vi "5. CSM Data Type.vi"() -> ()   [LabVIEW 2017]
doc: "### 5. CSM Data Type.vi\n\n#### Overview\n\nDemonstrates the data type descriptions recommended by CSM.\n\n#### Introduction\n\nIn the CSM framework, arguments can only be passed in the form of String types. To support various data types, data usually needs to go through a process of packing, transmission, and unpacking. For example, CSM internally provides support for the HEXSTR argument type, and users can also provide custom data type conversions via addons to suit their application scenarios.\n\nTo support different data types, you sometimes need to pass data type descriptions to handle logic branches for different data types at the decoding stage. This example demonstrates the data type description method recommended by CSM and the corresponding APIs."
uses:
  <vilib>/Utility/Data Type/Type Definitions/Data Type.ctl
  user.lib/_NEVSTOP/Communicable State Machine(CSM)/Utility/_support/CSM Data Type String to Enum(String).vi
  user.lib/_NEVSTOP/Communicable State Machine(CSM)/Communicable State Machine.lvlib
  <vilib>/Utility/Data Type/NI_Data Type.lvlib
panel:
  out "Array Dim 12":i32
  out "Secondary Type String 12":string
  out "Primary Type 12":T1
  out "Data Type String 12":string
  out "Array Dim 11":i32
  out "Secondary Type String 11":string
  out "Primary Type 11":T1
  out "Data Type String 11":string
  out "Array Dim 10":i32
  out "Secondary Type String 10":string
  out "Primary Type 10":T1
  out "Data Type String 10":string
  out "Array Dim 9":i32
  out "Secondary Type String 9":string
  out "Primary Type 9":T1
  out "Data Type String 9":string
  out "Array Dim 8":i32
  out "Secondary Type String 8":string
  out "Primary Type 8":T1
  out "Data Type String 8":string
  out "Array Dim 7":i32
  out "Secondary Type String 7":string
  out "Primary Type 7":T1
  out "Data Type String 7":string
  out "Array Dim 6":i32
  out "Secondary Type String 6":string
  out "Primary Type 6":T1
  out "Data Type String 6":string
  out "Array Dim 5":i32
  out "Secondary Type String 5":string
  out "Primary Type 5":T1
  out "Data Type String 5":string
  out "Array Dim 4":i32
  out "Secondary Type String 4":string
  out "Primary Type 4":T1
  out "Data Type String 4":string
  out "Array Dim 3":i32
  out "Secondary Type String 3":string
  out "Primary Type 3":T1
  out "Data Type String 3":string
  out "Array Dim 2":i32
  out "Secondary Type String 2":string
  out "Primary Type 2":T1
  out "Data Type String 2":string
  out "Data Type String":string
  out "Primary Type":T1
  out "Secondary Type String":string
  out "Array Dim":i32
  in  "Data 12":dbl[][](array[numeric])=[[3.12, 4.113, 2.3, 5.0, 5.0, 2.3, 4.11, 5.0]]
  in  "Data 11":T2(array[cluster])=[{"Name"="", "Child"={"Name"="ddd"}, "Bool"=FALSE}, {"Name"="ddd", "Child"={"Name"=""}, "Bool"=TRUE}]
  in  "Data 2":path=path "C:/ni-rt/data/a/2023.07.25"
  in  "Data 10":T3={"Name"="abc", "Child"={"Name"="ddd"}, "Bool"=FALSE}
  in  "Data 9":dbl[](array[numeric])=[3.12, 4.11, 5.0]
  in  "Data 8":enum16{"1 - aaaa", "2 - bbbb", "555 - ccccc"}(ring)=enum."555 - ccccc"
  in  "Data 7":enum16{"1 - aaaa", "2 - bbbb", "555 - ccccc"}(ring)=enum."555 - ccccc"
  in  "Data 6":enum16{"aaaa", "bbbb", "ccccc"}(ring)=enum."bbbb"
  in  "Data 5":dbl=3.1415926
  in  "Data 4":i32=66
  in  "Data 3":bool=TRUE
  in  "Data 1":string="abcd"
  # "#CSM-Example Overview\n\nDemonstrates the data type descriptions recommended by CSM."
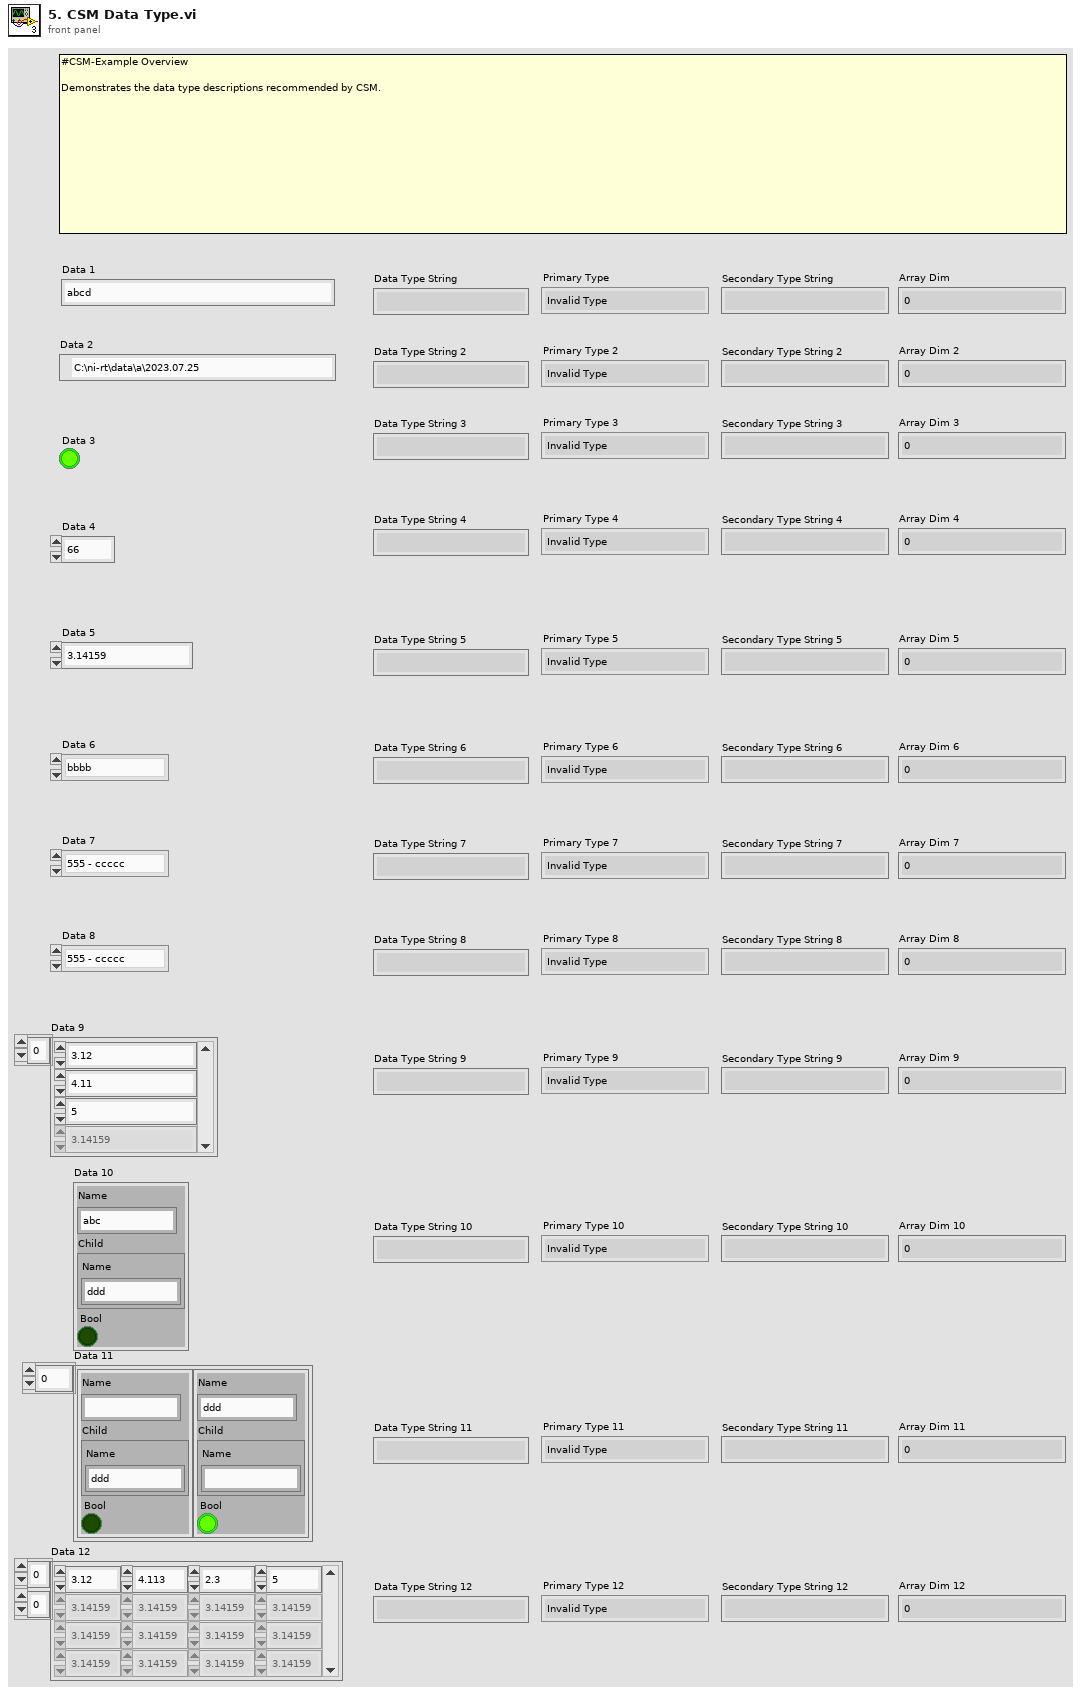
[diagram p1: front panel]
types:
  T1 = typedef "NI_Data Type.lvlib/Data Type.ctl" = enum8{"Invalid Type", "Void", "I8", "I16", "I32", "I64", "U8", "U16", "U32", "U64", "Single Float", "Double Float", "Extended Float", "Single Complex", "Double Complex", "Extended Complex", "Enum U8", "Enum U16", "Enum U32", "Enum U64", "Single Float With Unit", "Double Float With Unit", "Extended Float With Unit", "Single Complex with Unit", "Double Complex with Unit", "Extended Complex with Unit", "Boolean", "String", "Path", "Picture", "Tag", "Array", "Cluster", "Variant", "LV Variant", "Waveform", "Timestamp", "Digital Waveform", "Digital Data", "ExpressData", "Refnum", "External Data", "VI", "Poly VI", "LabVIEW Class Instance", "Fixed Point"}
  T2 = cluster{"Name":string, "Child":cluster{"Name":string}, "Bool":bool}[]
  T3 = cluster{"Name":string, "Child":cluster{"Name":string}, "Bool":bool}
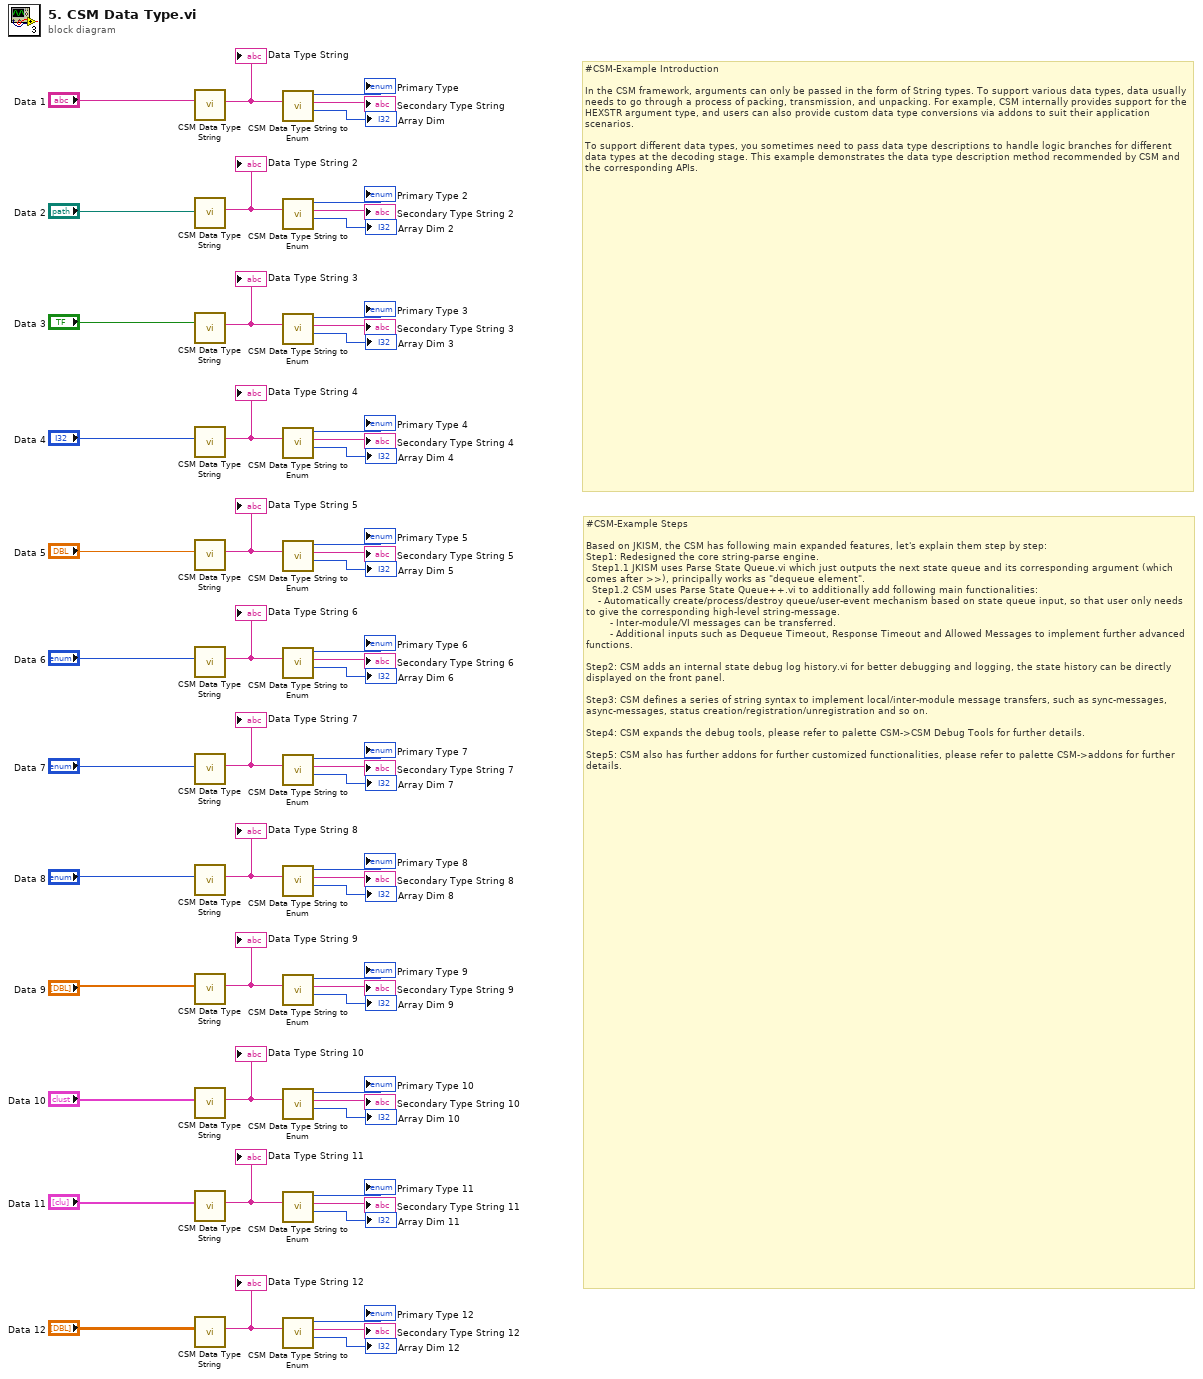
[diagram p0: block diagram]
diagram:
  # "#CSM-Example Steps\n\nBased on JKISM, the CSM has following main expanded features, let's explain them step by step:\nStep1: Redesigned the core string-parse engine.\n  Step1.1 JKISM uses Parse State Queue.vi which just outputs the next state queue and its corresponding argument (which comes after >>), principally works as \"dequeue element\".\n  Step1.2 CSM uses Parse State Queue++.vi to additionally add following main functionalities:\n    - Automatically create/process/destroy queue/user-event mechanism based on state queue input, so that user only needs to give the corresponding high-level string-message.\n        - Inter-module/VI messages can be transferred.\n        - Additional inputs such as Dequeue Timeout, Response Timeout and Allowed Messages to implement further advanced functions. \n\nStep2: CSM adds an internal state debug log history.vi for better debugging and logging, the state history can be directly displayed on the front panel.\n\nStep3: CSM defines a series of string syntax to implement local/inter-module message transfers, such as sync-messages, async-messages, status creation/registration/unregistration and so on.\n\nStep4: CSM expands the debug tools, please refer to palette CSM->CSM Debug Tools for further details.\n\nStep5: CSM also has further addons for further customized functionalities, please refer to palette CSM->addons for further details."
  # "#CSM-Example Introduction\n\nIn the CSM framework, arguments can only be passed in the form of String types. To support various data types, data usually needs to go through a process of packing, transmission, and unpacking. For example, CSM internally provides support for the HEXSTR argument type, and users can also provide custom data type conversions via addons to suit their application scenarios.\n\nTo support different data types, you sometimes need to pass data type descriptions to handle logic branches for different data types at the decoding stage. This example demonstrates the data type description method recommended by CSM and the corresponding APIs."
  n1 = call "CSM Data Type String.vi"("Data"="Data 1") -> ("Data Type String"=w60:string)  [unwired: 10 in]
  "Data Type String" <- w60
  n2 = call "CSM Data Type String.vi"("Data"="Data 2") -> ("Data Type String"=w52:string)  [unwired: 10 in]
  "Data Type String 2" <- w52
  n3 = call "CSM Data Type String.vi"("Data"="Data 3") -> ("Data Type String"=w50:string)  [unwired: 10 in]
  "Data Type String 3" <- w50
  n4 = call "CSM Data Type String.vi"("Data"="Data 4") -> ("Data Type String"=w42:string)  [unwired: 10 in]
  "Data Type String 4" <- w42
  n5 = call "CSM Data Type String.vi"("Data"="Data 5") -> ("Data Type String"=w40:string)  [unwired: 10 in]
  "Data Type String 5" <- w40
  n6 = call "CSM Data Type String.vi"("Data"="Data 6") -> ("Data Type String"=w32:string)  [unwired: 10 in]
  "Data Type String 6" <- w32
  n7 = call "CSM Data Type String.vi"("Data"="Data 7") -> ("Data Type String"=w30:string)  [unwired: 10 in]
  "Data Type String 7" <- w30
  n8 = call "CSM Data Type String.vi"("Data"="Data 8") -> ("Data Type String"=w22:string)  [unwired: 10 in]
  "Data Type String 8" <- w22
  n9 = call "CSM Data Type String.vi"("Data"="Data 9") -> ("Data Type String"=w20:string)  [unwired: 10 in]
  "Data Type String 9" <- w20
  n10 = call "CSM Data Type String.vi"("Data"="Data 10") -> ("Data Type String"=w12:string)  [unwired: 10 in]
  "Data Type String 10" <- w12
  n11 = call "CSM Data Type String.vi"("Data"="Data 11") -> ("Data Type String"=w10:string)  [unwired: 10 in]
  "Data Type String 11" <- w10
  n12 = call "CSM Data Type String.vi"("Data"="Data 12") -> ("Data Type String"=w2:string)  [unwired: 10 in]
  "Data Type String 12" <- w2
  n13 = call-poly "CSM Data Type String to Enum.vi"("Data Type String"=w60) -> ("Array Dim"=→"Array Dim":i32, "Secondary Type String"=→"Secondary Type String":string, "Primary Type"=→"Primary Type":T1)  [unwired: 8 in]
  n14 = call-poly "CSM Data Type String to Enum.vi"("Data Type String"=w52) -> ("Array Dim"=→"Array Dim 2":i32, "Secondary Type String"=→"Secondary Type String 2":string, "Primary Type"=→"Primary Type 2":T1)  [unwired: 8 in]
  n15 = call-poly "CSM Data Type String to Enum.vi"("Data Type String"=w50) -> ("Array Dim"=→"Array Dim 3":i32, "Secondary Type String"=→"Secondary Type String 3":string, "Primary Type"=→"Primary Type 3":T1)  [unwired: 8 in]
  n16 = call-poly "CSM Data Type String to Enum.vi"("Data Type String"=w42) -> ("Array Dim"=→"Array Dim 4":i32, "Secondary Type String"=→"Secondary Type String 4":string, "Primary Type"=→"Primary Type 4":T1)  [unwired: 8 in]
  n17 = call-poly "CSM Data Type String to Enum.vi"("Data Type String"=w40) -> ("Array Dim"=→"Array Dim 5":i32, "Secondary Type String"=→"Secondary Type String 5":string, "Primary Type"=→"Primary Type 5":T1)  [unwired: 8 in]
  n18 = call-poly "CSM Data Type String to Enum.vi"("Data Type String"=w32) -> ("Array Dim"=→"Array Dim 6":i32, "Secondary Type String"=→"Secondary Type String 6":string, "Primary Type"=→"Primary Type 6":T1)  [unwired: 8 in]
  n19 = call-poly "CSM Data Type String to Enum.vi"("Data Type String"=w30) -> ("Array Dim"=→"Array Dim 7":i32, "Secondary Type String"=→"Secondary Type String 7":string, "Primary Type"=→"Primary Type 7":T1)  [unwired: 8 in]
  n20 = call-poly "CSM Data Type String to Enum.vi"("Data Type String"=w22) -> ("Array Dim"=→"Array Dim 8":i32, "Secondary Type String"=→"Secondary Type String 8":string, "Primary Type"=→"Primary Type 8":T1)  [unwired: 8 in]
  n21 = call-poly "CSM Data Type String to Enum.vi"("Data Type String"=w20) -> ("Array Dim"=→"Array Dim 9":i32, "Secondary Type String"=→"Secondary Type String 9":string, "Primary Type"=→"Primary Type 9":T1)  [unwired: 8 in]
  n22 = call-poly "CSM Data Type String to Enum.vi"("Data Type String"=w12) -> ("Array Dim"=→"Array Dim 10":i32, "Secondary Type String"=→"Secondary Type String 10":string, "Primary Type"=→"Primary Type 10":T1)  [unwired: 8 in]
  n23 = call-poly "CSM Data Type String to Enum.vi"("Data Type String"=w10) -> ("Array Dim"=→"Array Dim 11":i32, "Secondary Type String"=→"Secondary Type String 11":string, "Primary Type"=→"Primary Type 11":T1)  [unwired: 8 in]
  n24 = call-poly "CSM Data Type String to Enum.vi"("Data Type String"=w2) -> ("Array Dim"=→"Array Dim 12":i32, "Secondary Type String"=→"Secondary Type String 12":string, "Primary Type"=→"Primary Type 12":T1)  [unwired: 8 in]
